vi "createWaveData.vi"(8 "error in (no error)":errorcluster, 9 "samplesPerChunkPerChannel":i32, 10 "segementData":T1(array[cluster]), 11 "SoundDeviceData in":refnum<class "SoundDeviceData.lvclass">) -> (0 "error out":errorcluster, 2 "Path":path, 3 "SoundDeviceData out":refnum<class "SoundDeviceData.lvclass">)   [LabVIEW 2009, in "DataMappers.lvlib" / "SoundDeviceData.lvclass"]
uses:
  SoundDeviceData.lvclass
  DatabaseHelpers/Database Objects/Channel/Channel.lvclass
  SoundDeviceData.lvclass/SoundDeviceData.ctl
  <vilib>/sound2/lvsound2.llb/Sound File Write Open.vi
  <vilib>/sound2/lvsound2.llb/Sound File Write (DBL).vi
  Filing/FileNeologist/FileNeologist.lvclass
  Filing.lvlib
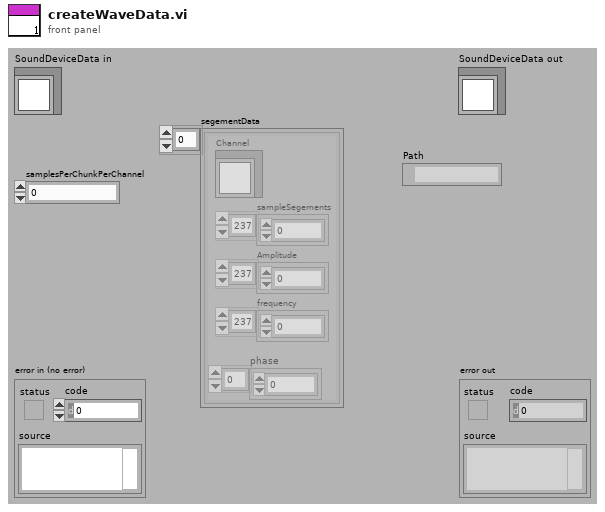
[diagram p1: front panel]
types:
  T1 = cluster{"Channel":refnum<class "Channel.lvclass">, "sampleSegements":dbl[], "Amplitude":dbl[], "frequency":dbl[], "phase":dbl[]}[]
  T2 = cluster{"Channel":refnum<class "Channel.lvclass">, "sampleSegements":dbl[], "Amplitude":dbl[], "frequency":dbl[], "phase":dbl[]}
  T3 = typedef "Sound File Refnum.ctl" = refnum<file>
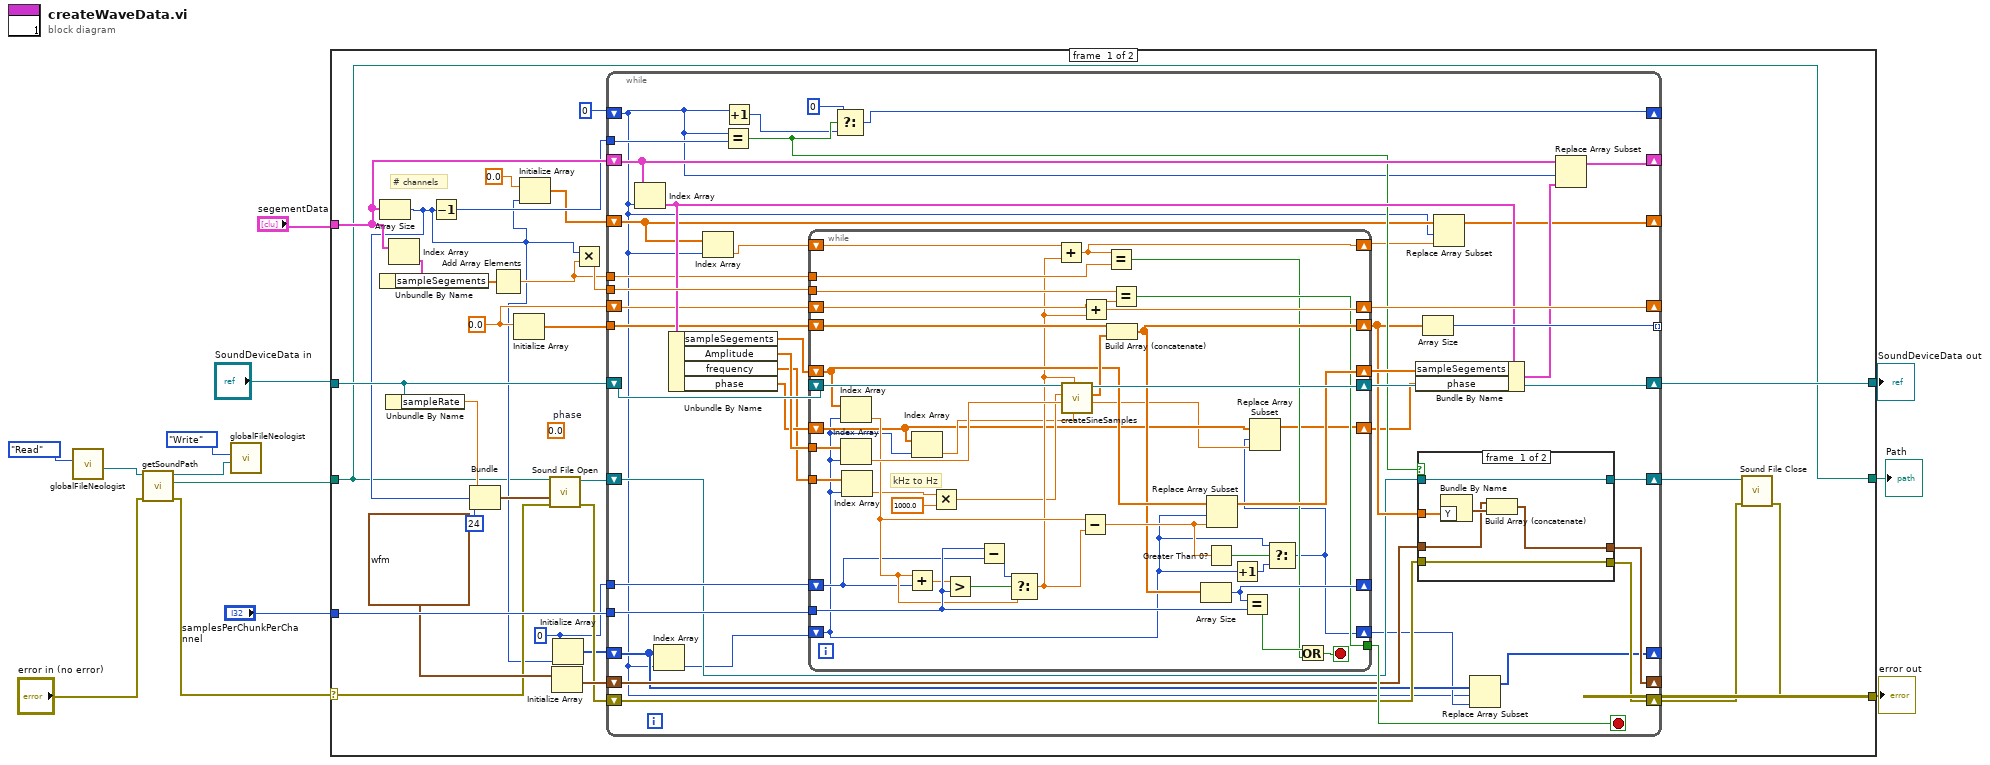
[diagram p0: block diagram]
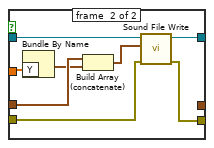
[diagram p2: hidden frame]
diagram:
  n1 = call "globalFileNeologist.vi"("Action"=enum16{"Write", "Read"}."Read") -> ("FileNeologist out"=w8:refnum<class "FileNeologist.lvclass">)  [unwired: 10 in]
  n2 = call "getSoundPath.vi"("error in (no error)"="error in (no error)", "FileNeologist in"=w8) -> ("error out"=w2:errorcluster, "Path"=w4:path, "FileNeologist out"=w5:refnum<class "FileNeologist.lvclass">)  [unwired: 7 in]
  n3 = call "globalFileNeologist.vi"("FileNeologist in"=w5, "Action"=enum16{"Write", "Read"}."Write") -> ()  [unwired: 9 in, 1 out]
  n4 = case shown="No Error" w2 {
    selector: w2 -> [w35 w140]
    tunnel: [w26 w140] -> w13
    tunnel: [w39 w139] -> w11
    tunnel: "SoundDeviceData in" -> [w21 w139]
    tunnel: "segementData" -> [w33 _]
    tunnel: "samplesPerChunkPerChannel" -> [w42 _]
    tunnel: w4 -> [w14 _]
    tunnel: [w14 _] -> w1
    frame #0 {
      (unwired) 0.0  # phase
      w40 = 0.0
      w24 = 0
      # "# channels"
      n5 = Array Size(array=w33) -> (size(s)=w15:i32)
      n6 = Unbundle By Name(w21) -> ("sampleRate"=w20:dbl)
      n7 = Index Array(array=w33) -> (element=w32:T2)  [unwired: 1 in]
      n8 = Unbundle By Name(w32) -> ("sampleSegements"=w31:dbl[])
      n9 = Decrement(x=w15) -> (x-1=w23:i32)
      n10 = Bundle("sampleRate"=w20, w15, 24) -> (w22:cluster{"sampleRate":dbl, i32, i32})  [unwired: 1 in]
      n11 = Add Array Elements(numeric array=w31) -> (sum=w19:dbl)
      n12 = Initialize Array(w40) -> (w18:dbl[])  [unwired: 1 in]
      n13 = Initialize Array(0.0, w15) -> (w17:dbl[])
      n14 = call-poly <vilib>:"Sound File Open.vi"("error in (no error)"=w35, "sound format"=w22, "path"=w14) -> ("error out"=w34:errorcluster, "sound file refnum"=w36:T3)  [unwired: 7 in]
      n15 = Initialize Array(waveform(dbl) {"t0"=timestamp(0 s since 1904-01-01), "dt"=1.0, "Y"=[]}) -> (w37:waveform(dbl)[])  [unwired: 1 in]
      n16 = Initialize Array(w24, w15) -> (w25:i32[])
      n17 = Multiply(x=w15, y=w19) -> (x*y=w30:dbl)
      n18 = while {
        shift-right: [w83] -> w39
        shift-left: w21 -> [w84]
        tunnel: w42 -> [w82]
        tunnel: w24 -> [w81]
        tunnel: w18 -> [w69]
        tunnel: [w80] -> _ mode=indexing
        tunnel: w30 -> [w77]
        shift-right: [w79] -> _
        shift-left: w40 -> [w51]
        shift-right: [w68] -> _
        shift-left: w33 -> [w67]
        tunnel: w23 -> [w76]
        shift-right: [w74] -> _
        shift-left: 0 -> [w48]
        shift-right: [w62] -> _
        shift-left: w37 -> [w63]
        shift-right: [w61] -> w28
        shift-left: w36 -> [w59]
        shift-right: [w57] -> w27
        shift-left: w34 -> [w58]
        shift-right: [w53] -> _
        shift-left: w25 -> [w55]
        tunnel: w19 -> [w52]
        shift-right: [w46] -> _
        shift-left: w17 -> [w49]
        stop <- w78 stop-if-true
        n19 = Index Array(array=w67, index=w48) -> (element=w72:T2)
        n20 = Index Array(array=w55, index=w48) -> (element=w56:i32)
        n21 = Unbundle By Name(w72) -> ("sampleSegements"=w73:dbl[], "Amplitude"=w70:dbl[], "frequency"=w44:dbl[], "phase"=w45:dbl[])
        n22 = Index Array(array=w49, index=w48) -> (element=w50:dbl)
        n23 = Equal?(x=w48, y=w76) -> (x = y?=w65:bool)
        n24 = Increment(x=w48) -> (x+1=w60:i32)
        n25 = while {
          shift-right: [w99] -> w54
          shift-left: w56 -> [w100]
          tunnel: w82 -> [w128]
          tunnel: w70 -> [w135]
          tunnel: w44 -> [w134]
          shift-right: [w115] -> w64
          shift-left: w69 -> [w132]
          shift-right: [w130] -> _
          shift-left: w81 -> [w117]
          shift-right: [w124] -> w71
          shift-left: w73 -> [w125]
          shift-right: [w113] -> w79
          shift-left: w51 -> [w119]
          tunnel: w77 -> [w118]
          tunnel: [w109] -> w78
          shift-right: [w137] -> w83
          shift-left: w84 -> [w138]
          tunnel: w52 -> [w114]
          shift-right: [w111] -> w47
          shift-left: w50 -> [w112]
          shift-right: [w101] -> w43
          shift-left: w45 -> [w103]
          stop <- w116 stop-if-true
          # "kHz to Hz"
          n26 = Index Array(array=w125, index=w100) -> (element=w120:dbl)
          n27 = Index Array(array=w135, index=w100) -> (element=w133:dbl)
          n28 = Index Array(array=w134, index=w100) -> (element=w107:dbl)
          n29 = Add(x=w120, y=w117) -> (x+y=w126:dbl)
          n30 = Index Array(array=w103, index=w100) -> (element=w104:dbl)
          n31 = Multiply(x=w107, y=1000.0) -> (x*y=w105:dbl)
          n32 = Greater?(x=w126, y=w128) -> (0:w129:bool)
          n33 = Subtract(x=w128, y=w117) -> (x-y=w127:i32)
          n34 = Select(t=w127, s=w129, f=w120) -> (s? t:f=w110:dbl)
          n35 = Add(x=w112, y=w110) -> (x+y=w111:dbl)
          n36 = call "createSineSamples.vi"("phase"=w104, "samples"=w110, "amplitude"=w133, "freq"=w105, "SoundDeviceData in"=w138) -> ("phase out"=w102:dbl, "sine wave"=w131:dbl[], "SoundDeviceData out"=w137:refnum<class "SoundDeviceData.lvclass">)  [unwired: 3 in, 1 out]
          n37 = Subtract(x=w120, y=w110) -> (x-y=w123:dbl)
          n38 = Add(x=w119, y=w110) -> (x+y=w113:dbl)
          n39 = Equal?(x=w111, y=w114) -> (x = y?=w108:bool)
          n40 = Build Array (concatenate)(w132, w131) -> (w115:dbl[])
          n41 = Equal?(x=w118, y=w113) -> (x = y?=w109:bool)
          n42 = Array Size(array=w115) -> (size(s)=w130:i32)
          n43 = Greater Than 0?(x=w123) -> (x > 0?=w122:bool)
          n44 = Replace Array Subset(array=w125, new element=w123, index=w100) -> (w124:dbl[])
          n45 = Increment(x=w100) -> (x+1=w121:i32)
          n46 = Equal?(x=w130, y=w128) -> (x = y?=w136:bool)
          n47 = Select(t=w100, s=w122, f=w121) -> (s? t:f=w99:i32)
          n48 = Replace Array Subset(array=w103, new element=w102, index=w99) -> (w101:dbl[])
          n49 = Or(x=w136, y=w108) -> (x .or. y?=w116:bool)
        }
        n50 = Select(t=0, s=w65, f=w60) -> (s? t:f=w74:i32)
        n51 = Bundle By Name(cluster=w72, "sampleSegements"=w71, "phase"=w43) -> (w66:T2)
        n52 = case shown="True" w65 {
          tunnel: w64 -> [w90 w97]
          tunnel: w63 -> [w87 w98]
          tunnel: [w88 _] -> w62
          tunnel: w59 -> [w86 w94]
          tunnel: [w86 w93] -> w61
          tunnel: w58 -> [w85 w92]
          tunnel: [w85 w91] -> w57
          frame #0 {
            n53 = Bundle By Name("Y"=w90) -> (w89:waveform(dbl))  [unwired: 1 in]
            n54 = Build Array (concatenate)(w87, w89) -> (w88:waveform(dbl)[])
          }
          frame #1 {
            n55 = Bundle By Name("Y"=w97) -> (w96:waveform(dbl))  [unwired: 1 in]
            n56 = Build Array (concatenate)(w98, w96) -> (w95:waveform(dbl)[])
            n57 = call-poly <vilib>:"Sound File Write.vi"("error in (no error)"=w92, "data"=w95, "sound file refnum"=w94) -> ("error out"=w91:errorcluster, "sound file refnum out"=w93:T3)  [unwired: 7 in]
          }
        }
        n58 = Array Size(array=w64) -> (size(s)=w80:i32)
        n59 = Replace Array Subset(array=w49, new element=w47, index=w48) -> (w46:dbl[])
        n60 = Replace Array Subset(array=w55, new element=w54, index=w48) -> (w53:i32[])
        n61 = Replace Array Subset(array=w67, new element=w66, index=w48) -> (w68:T1)
      }
      n62 = call <vilib>:"Sound File Close.vi"("error in (no error)"=w27, "sound file refnum"=w28) -> ("error out"=w26:errorcluster)  [unwired: 9 in]
    }
    frame #1 {
    }
  }
  "error out" <- w13
  "SoundDeviceData out" <- w11
  "Path" <- w1
